vi "LJUD_eAddGoGet.vi"(0 "Handle In":i32, 1 "aIOTypes":i32[](array[numeric]), 2 "aChannels":i32[](array[numeric]), 5 "Values Write":dbl[](array[numeric]) format="%.2f", 7 "ax1s":i32[](array[numeric]), 9 "NumRequests":i32, 11 "error in":errorcluster) -> (4 "Handle Out":i32, 6 "Values Read":dbl[](array[numeric]) format="%.2f", 8 "aRequestErrors":i32[](array[numeric]), 10 "GoError":i32, 14 "aResultErrors":i32[](array[numeric]), 15 "error out":errorcluster)   [LabVIEW 2021]
doc: "This is a call to eAddGoGet from the UD libary. By passing arrays of requests\nand results this function combines add-add-go-get-get into a single function\ncall.\n\nIn LabVIEW an alternative way to do multiple requests and results with a single\nsub-VI is the utility AddS-Go-Get.vi. The utility VI has better/easier error handling\nand is normally preferred in LabVIEW, but eAddGoGet is a single call to the UD\ndriver so often preferred if you will have parallel driver calls within the same thread.\n\nThis is a traditional technique UD function ... Add-Add-Go-Get-Get. See Section 4.1\nof the device's datasheet for more information.\n\nIOType specifies what sort of action will be performed. The other inputs depend\non the IOType. See the pseudocode in Section 4.3 for info."
uses:
  labjackud.dll
panel:
  # "This is a call to eAddGoGet from the UD libary.  By passing arrays of requests\nand results this function combines add-add-go-get-get into a single function\ncall.\n\nIn LabVIEW an alternative way to do multiple requests and results with a single\nsub-VI is the utility AddS-Go-Get.vi.  The utility VI has better/easier error handling\nand is normally preferred in LabVIEW, but eAddGoGet is a single call to the UD\ndriver so often preferred if you will have parallel driver calls within the same thread.\n\nThis is a traditional technique UD function ... Add-Add-Go-Get-Get. See Section 4.1\nof the device's datasheet for more information.\n\nIOType specifies what sort of action will be performed.  The other inputs depend\non the IOType.  See the pseudocode in Section 4.3 for info."
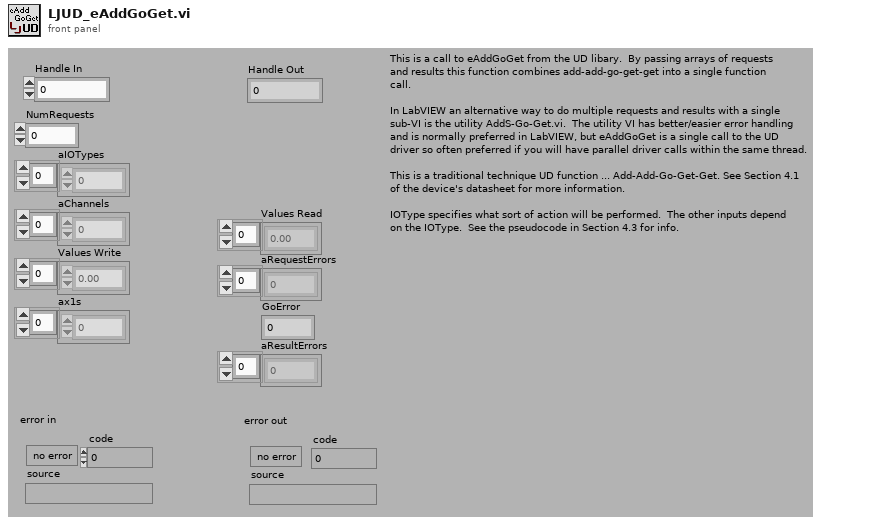
[diagram p1: front panel]
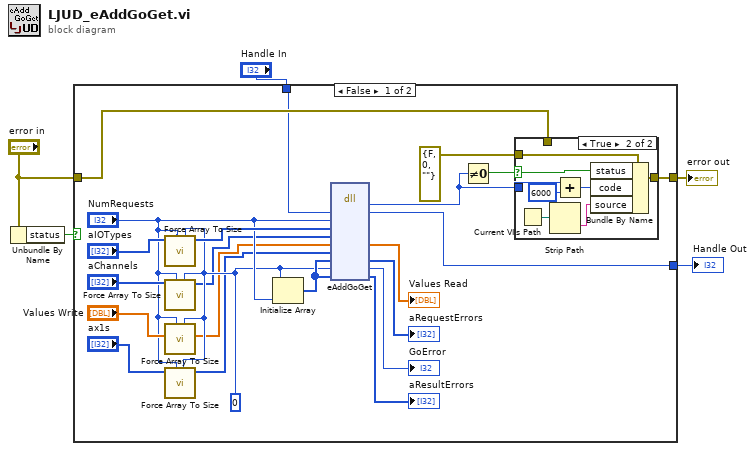
[diagram p0: block diagram]
diagram:
  n1 = Unbundle By Name("error in") -> ("status"=w4:bool)
  n2 = case shown="False" w4 {
    tunnel: [w24 w38] -> w5
    tunnel: "error in" -> [w23 w38]
    tunnel: "Handle In" -> [w17 w37]
    tunnel: [w16 w37] -> w1
    frame False {
      w9 = 0 ("GoError")
      n3 = call "Force Array To Size.vi"("Default Value"=w9, "# Elements"="NumRequests", "I32 Array In"="aIOTypes") -> ("I32 Array Out"=w11:i32[])  [unwired: 5 in, 3 out]
      n4 = call "Force Array To Size.vi"("Default Value"=w9, "# Elements"="NumRequests", "I32 Array In"="aChannels") -> ("I32 Array Out"=w8:i32[])  [unwired: 5 in, 3 out]
      n5 = call "Force Array To Size.vi"("Default Value"=w9, "# Elements"="NumRequests", "DBL Array In"="Values Write") -> ("DBL Array Out"=w7:dbl[])  [unwired: 5 in, 3 out]
      n6 = call "Force Array To Size.vi"("Default Value"=w9, "# Elements"="NumRequests", "I32 Array In"="ax1s") -> ("I32 Array Out"=w6:i32[])  [unwired: 5 in, 3 out]
      n7 = Initialize Array(w9, "NumRequests") -> (w22:i32[])
      n8 = dll-call lib="labjackud.dll" fn="eAddGoGet"("Handle"=w17, "NumRequests"="NumRequests", "aIOTypes"=w11, "aChannels"=w8, "aValues"=w7, "ax1s"=w6, "aRequestErrors"=w22, "GoError"=w9, "aResultErrors"=w22) -> (w25:i32, "Handle"=w16:i32, "aValues"=→"Values Read":dbl[], "aRequestErrors"=→"aRequestErrors":i32[], "GoError"=→"GoError":i32, "aResultErrors"=→"aResultErrors":i32[])  [unwired: 7 in, 2 out]
      n9 = Not Equal To 0?(x=w25) -> (x != 0?=w26:bool)
      n10 = case shown="True" w26 {
        selector: w26 -> [_ w35]
        tunnel: [w28 w36] -> w24
        tunnel: errorcluster {"status"=FALSE, "code"=0, "source"=""} ("error IO") -> [_ w34]
        tunnel: w25 -> [_ w30]
        tunnel: w23 -> [w28 _]
        frame False {
        }
        frame True {
          n11 = Current VI's Path() -> (path=w32:path)
          n12 = Strip Path(path=w32) -> (name=w33:string)  [unwired: 1 out]
          n13 = Add(x=w30, y=6000) -> (x+y=w31:i32)
          n14 = Bundle By Name(cluster=w34, "status"=w35, "code"=w31, "source"=w33) -> (w36:errorcluster)
        }
      }
    }
    frame True {
    }
  }
  "error out" <- w5
  "Handle Out" <- w1
